vi "simulatorCommandPacketErForce.vi"(5 "degubBall":bool=TRUE, 6 "replaceRobots":bool, 7 "replaceBall":bool=TRUE, 10 "Ball":refnum<class "Ball.lvclass">, 11 "grSIM replacement":T1) -> (3 "Array":u8[](array[numeric]))   [LabVIEW 2023, in "Communication.lvclass"]
uses:
  Communication.lvclass
  Controls/grSimReplacement.ctl
  grSim Packet Command UDP Test Folder/grSim/grSim RobotReplacement.ctl
  grSim Packet Command UDP Test Folder/grSim/grSim_BallReplacement.ctl
  Ball_class/Ball.lvclass
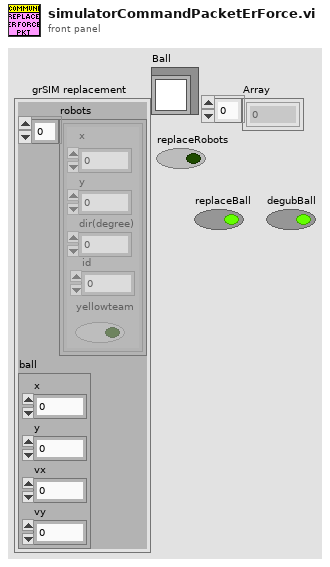
[diagram p1: front panel]
types:
  T1 = typedef "grSimReplacement.ctl" = cluster{"robots":T2[], "ball":T3}
  T2 = typedef "grSim RobotReplacement.ctl" = cluster{"x":dbl, "y":dbl, "dir(degree)":dbl, "yellowteam":bool, "id":u32}
  T3 = typedef "grSim_BallReplacement.ctl" = cluster{"x":dbl, "y":dbl, "vx":dbl, "vy":dbl}
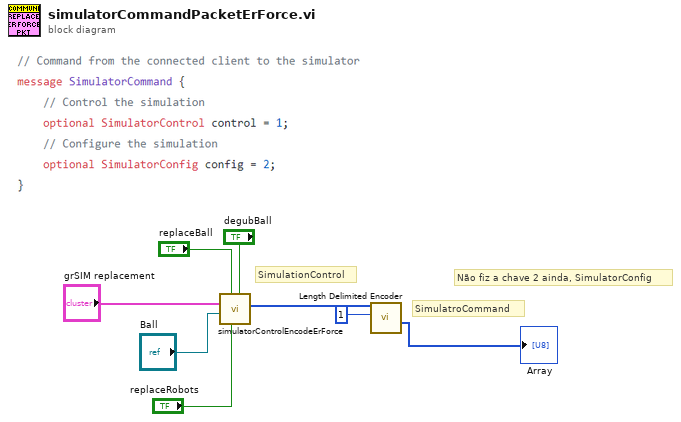
[diagram p0: block diagram]
diagram:
  # "SimulatroCommand"
  # "SimulationControl"
  # "Não fiz a chave 2 ainda, SimulatorConfig"
  n1 = call "simulatorControlEncodeErForce.vi"("degubBall"="degubBall", "replaceRobots"="replaceRobots", "replaceBall"="replaceBall", "Ball"="Ball", "grSIM replacement"="grSIM replacement") -> ("SimulatorControlArray"=w6:u8[])  [unwired: 4 in, 2 out]
  n2 = call "Length Delimited Encoder.vi"("Key"=u32 1, "Array In to be added"=w6) -> ("Array"=→"Array":u8[])  [unwired: 9 in]
